vi "Test.vi"(0 "Call Context":T9, 5 "Test Controls":T3 {"Slider" scale=-1.0..1.0}) -> (1 "SubState 0":T2=enum."driver control", 2 "SubState 4":T2, 3 "Loop 0 Data":T7, 4 "SubState 1":T2, 6 "Loop 1 Data":T6, 10 "SubState 2":T2, 11 "SubState 5":T8, 12 "Loop 3 Data":T4, 13 "Loop 4 Data":T1, 14 "SubState 3":T2, 15 "Loop 2 Data":T5)   [LabVIEW 2013]
uses:
  typedefs/state machine/subStates.ctl
  <vilib>/Rock Robotics/WPI/DriverStation/WPI_DriverStationDerivedRobotMode.ctl
  typedefs/state machine/singleUseSubstate.ctl
  typedefs/loop datatypes/Loop 0 Datatype.ctl
  typedefs/loop datatypes/Loop 1 Datatype.ctl
  typedefs/loop datatypes/Loop 2 Datatype.ctl
  typedefs/loop datatypes/Loop 3 Datatype.ctl
  typedefs/test/test controls.ctl
  typedefs/loop datatypes/Loop 4 Datatype.ctl
  typedefs/fg_getset.ctl
  <vilib>/Rock Robotics/WPI/Joystick/WPI_JoystickGetSetRefNum.vi
panel:
  out "Compressor":bool
  out "JS Axis-Y 3":dbl
  out "JS Axis-X 3":dbl
  out "JS Axis-Y 2":dbl
  out "JS Axis-X 2":dbl
  out "UDB":bool
  out "JS Axis-X":dbl
  out "JS Axis-Y":dbl
  out "Exit Value":i32=-1
  # "Test Loop Data and Substates"
  # "Drive Loop"
  # "Loop 1"
  # "Loop 2"
  # "Loop 3"
  # "Loop 4"
  # "Pneumatics Loop"
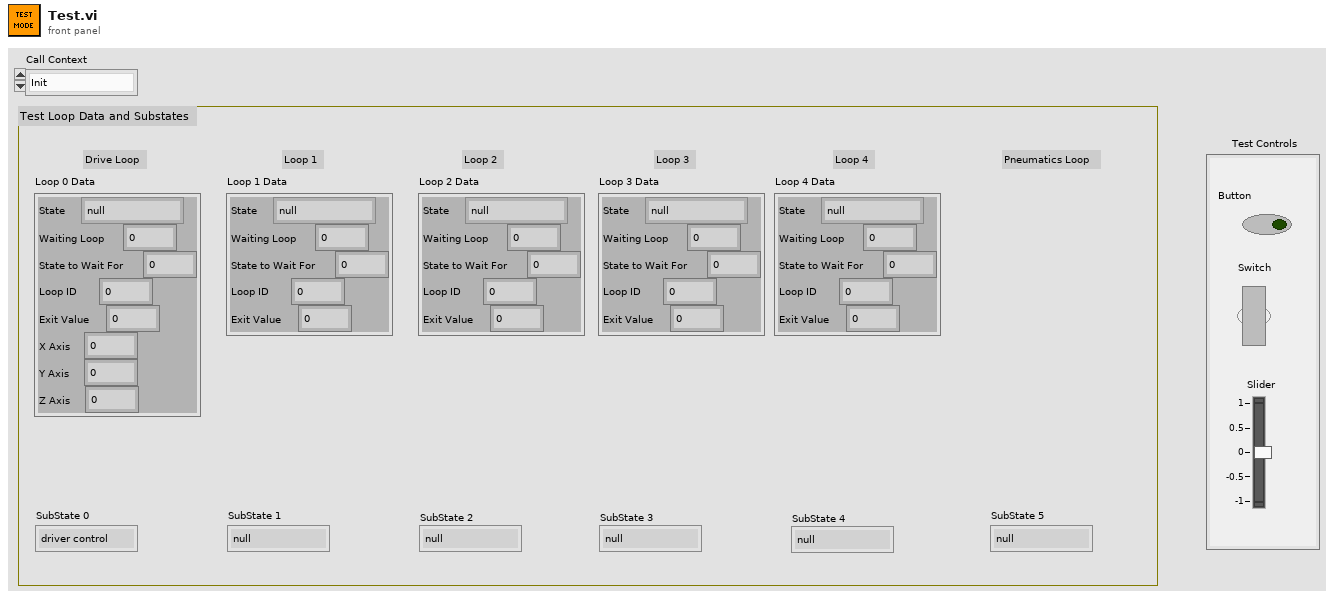
[diagram p1: front panel]
types:
  T1 = typedef "Loop 4 Datatype.ctl" = cluster{"State":T2, "Waiting Loop":i32, "State to Wait For":i32, "Loop ID":i32, "Exit Value":i32}
  T2 = typedef "subStates.ctl" = enum16{"null", "wait", "driver control", "auto", "manual override", "hold position", "rotate", "test", "end"}
  T3 = typedef "test controls.ctl" = cluster{"Button":bool, "Switch":bool, "Slider":dbl}
  T4 = typedef "Loop 3 Datatype.ctl" = cluster{"State":T2, "Waiting Loop":i32, "State to Wait For":i32, "Loop ID":i32, "Exit Value":i32}
  T5 = typedef "Loop 2 Datatype.ctl" = cluster{"State":T2, "Waiting Loop":i32, "State to Wait For":i32, "Loop ID":i32, "Exit Value":i32}
  T6 = typedef "Loop 1 Datatype.ctl" = cluster{"State":T2, "Waiting Loop":i32, "State to Wait For":i32, "Loop ID":i32, "Exit Value":i32}
  T7 = typedef "Loop 0 Datatype.ctl" = cluster{"State":T2, "Waiting Loop":i32, "State to Wait For":i32, "Loop ID":i32, "Exit Value":i32, "X Axis":dbl, "Y Axis":dbl, "Z Axis":dbl}
  T8 = typedef "singleUseSubstate.ctl" = enum16{"null", "wait", "shift high", "shift low", "end"}
  T9 = typedef "WPI_DriverStationDerivedRobotMode.ctl" = enum16{"Init", "Execute", "Stop"}
  T10 = typedef "fg_getset.ctl" = enum16{"Get", "Set"}
  T11 = typedef "WPI_JoystickDevRef.ctl" = cluster{"Device":T12}
  T12 = typedef "WPI_JoystickDeviceEnum.ctl" = enum16{"USB 1", "USB 2", "USB 3", "USB 4", "Kinect 1", "Kinect 2"}
  T13 = cluster{"axis 1 (x)":dbl, "axis 2 (y)":dbl, "axis 3 (throttle)":dbl, "axis 4":dbl, "axis 5":dbl, "axis 6":dbl}
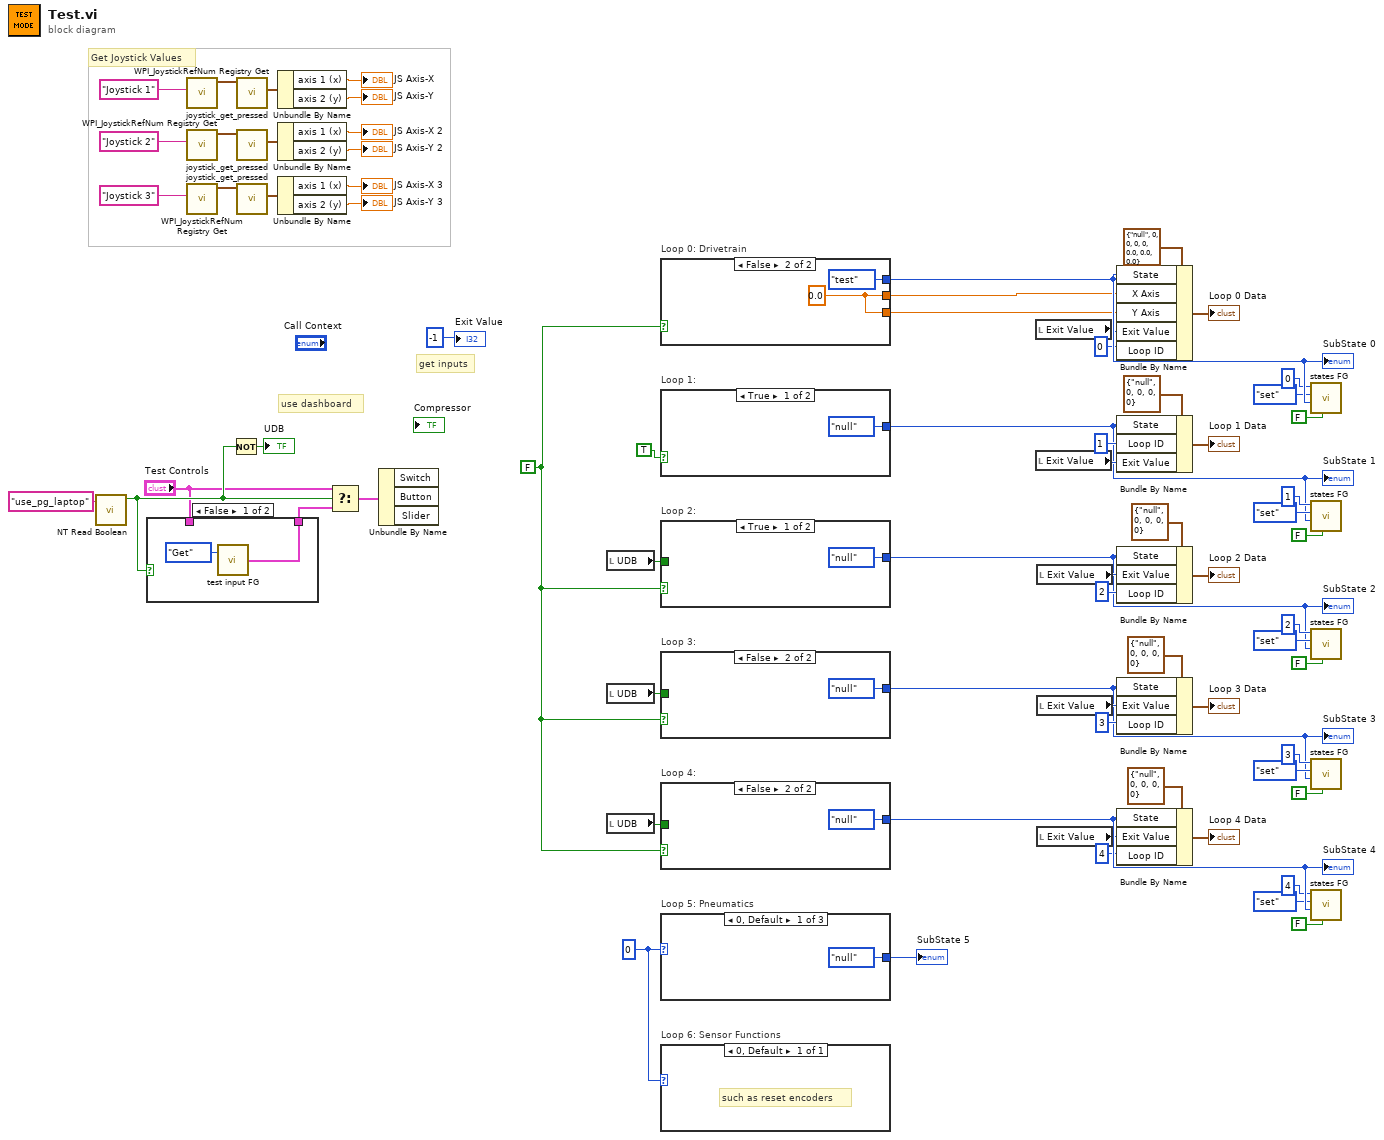
[diagram p0: block diagram]
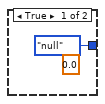
[diagram p2: hidden frame]
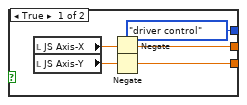
[diagram p4: hidden frame]
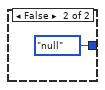
[diagram p5: hidden frame]
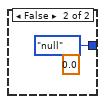
[diagram p6: hidden frame]
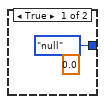
[diagram p7: hidden frame]
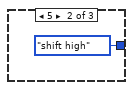
[diagram p8: hidden frame]
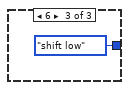
[diagram p9: hidden frame]
diagram:
  w1 = 0 ("Button Pressed")
  w6 = FALSE
  # "use dashboard"
  # "get inputs"
  # "Get Joystick Values"
  n1 = call <vilib>:"NT Read Boolean.vi"("Name"="use_pg_laptop") -> ("Boolean"=w31:bool)  [unwired: 9 in, 1 out]
  n2 = case shown="False" w31 {
    tunnel: [w73 w74] -> w29
    tunnel: "Test Controls" -> [_ w74]
    frame False {
      n3 = call "test input FG.vi"("Menu"=fg_getset."Get") -> ("Test Controls Out"=w73:T3)  [unwired: 1 in]
    }
    frame True {
    }
  }
  n4 = call <vilib>:"WPI_JoystickRefNum Registry Get.vi"("refnum name"="Joystick 1") -> ("JoystickDevRef"=w65:T11)  [unwired: 9 in, 1 out]
  n5 = call <vilib>:"WPI_JoystickRefNum Registry Get.vi"("refnum name"="Joystick 2") -> ("JoystickDevRef"=w25:T11)  [unwired: 9 in, 1 out]
  n6 = call <vilib>:"WPI_JoystickRefNum Registry Get.vi"("refnum name"="Joystick 3") -> ("JoystickDevRef"=w22:T11)  [unwired: 9 in, 1 out]
  n7 = Not(x=w31) -> (.not. x?=→"UDB":bool)
  n8 = call "joystick_get_pressed.vi"("JoystickDevRef"=w65) -> ("Axes"=w63:T13)  [unwired: 3 in, 3 out]
  n9 = call "joystick_get_pressed.vi"("JoystickDevRef"=w25) -> ("Axes"=w26:T13)  [unwired: 3 in, 3 out]
  n10 = call "joystick_get_pressed.vi"("JoystickDevRef"=w22) -> ("Axes"=w21:T13)  [unwired: 3 in, 3 out]
  n11 = Unbundle By Name(w63) -> ("axis 1 (x)"=→"JS Axis-X":dbl, "axis 2 (y)"=→"JS Axis-Y":dbl)
  n12 = Unbundle By Name(w26) -> ("axis 1 (x)"=→"JS Axis-X 2":dbl, "axis 2 (y)"=→"JS Axis-Y 2":dbl)
  n13 = Unbundle By Name(w21) -> ("axis 1 (x)"=→"JS Axis-X 3":dbl, "axis 2 (y)"=→"JS Axis-Y 3":dbl)
  n14 = Select(t="Test Controls", s=w31, f=w29) -> (s? t:f=w32:T3)
  n15 = Unbundle By Name(w32) -> ()  [unwired: 3 out]
  n16 = local read "UDB"() -> (w17:bool)
  n17 = local read "UDB"() -> (w16:bool)
  n18 = local read "UDB"() -> (w12:bool)
  n19 = case "Loop 0: Drivetrain" shown="False" w6 {
    tunnel: [w75 w80] -> w34
    tunnel: [subStates."driver control" ("State") subStates."test" ("State")] -> w71
    tunnel: [w76 w80] -> w35
    frame True {
      n20 = local read "JS Axis-X"() -> (w78:dbl)
      n21 = local read "JS Axis-Y"() -> (w77:dbl)
      n22 = Negate(x=w78) -> (-x=w76:dbl)
      n23 = Negate(x=w77) -> (-x=w75:dbl)
    }
    frame False {
      w80 = 0.0 ("JS Axis-X")
    }
  }
  "SubState 0" <- w71
  n24 = case "Loop 1:" shown="True" TRUE {
    tunnel: [subStates."null" ("State") subStates."null" ("State")] -> w42
    frame True {
    }
    frame False {
    }
  }
  "SubState 1" <- w42
  n25 = case "Loop 2:" shown="True" w6 {
    tunnel: [subStates."null" ("State") subStates."null" ("State")] -> w14
    tunnel: w17 -> [_ _]
    frame True {
    }
    frame False {
      (unwired) 0.0 ("Belts")
    }
  }
  "SubState 2" <- w14
  n26 = case "Loop 3:" shown="False" w6 {
    tunnel: [subStates."null" ("State") subStates."null" ("State")] -> w15
    tunnel: w16 -> [_ _]
    frame True {
      (unwired) 0.0 ("Arm")
    }
    frame False {
    }
  }
  "SubState 3" <- w15
  n27 = case "Loop 4:" shown="False" w6 {
    tunnel: [subStates."null" ("State") subStates."null" ("State")] -> w13
    tunnel: w12 -> [_ _]
    frame True {
      (unwired) 0.0 ("Arm")
    }
    frame False {
    }
  }
  "SubState 4" <- w13
  n28 = case "Loop 5: Pneumatics" shown="0, Default" w1 {
    tunnel: [singleUseSubstate."null" ("SubState 4") singleUseSubstate."shift high" ("SubState 4") singleUseSubstate."shift low" ("SubState 4")] -> w70
    frame 0, Default {
    }
    frame 5 {
    }
    frame 6 {
    }
  }
  "SubState 5" <- w70
  n29 = case "Loop 6: Sensor Functions" shown="0, Default" w1 {
    frame 0, Default {
      # "such as reset encoders"
    }
  }
  n30 = local read "Exit Value"() -> (w39:i32)
  n31 = local read "Exit Value"() -> (w50:i32)
  n32 = local read "Exit Value"() -> (w54:i32)
  n33 = local read "Exit Value"() -> (w64:i32)
  n34 = local read "Exit Value"() -> (w7:i32)
  n35 = Bundle By Name(cluster=T7 {"State"=enum."null", "Waiting Loop"=0, "State to Wait For"=0, "Loop ID"=0, "Exit Value"=0, "X Axis"=0.0, "Y Axis"=0.0, "Z Axis"=0.0} ("Loop 0 Data"), "State"=w71, "X Axis"=w35, "Y Axis"=w34, "Exit Value"=w39, "Loop ID"=0) -> (→"Loop 0 Data":T7)
  n36 = Bundle By Name(cluster=T6 {"State"=enum."null", "Waiting Loop"=0, "State to Wait For"=0, "Loop ID"=0, "Exit Value"=0} ("Loop 1 Data"), "State"=w42, "Loop ID"=1, "Exit Value"=w50) -> (→"Loop 1 Data":T6)
  n37 = Bundle By Name(cluster=T5 {"State"=enum."null", "Waiting Loop"=0, "State to Wait For"=0, "Loop ID"=0, "Exit Value"=0} ("Loop 2 Data"), "State"=w14, "Exit Value"=w54, "Loop ID"=2) -> (→"Loop 2 Data":T5)
  n38 = Bundle By Name(cluster=T4 {"State"=enum."null", "Waiting Loop"=0, "State to Wait For"=0, "Loop ID"=0, "Exit Value"=0} ("Loop 3 Data"), "State"=w15, "Exit Value"=w64, "Loop ID"=3) -> (→"Loop 3 Data":T4)
  n39 = Bundle By Name(cluster=T1 {"State"=enum."null", "Waiting Loop"=0, "State to Wait For"=0, "Loop ID"=0, "Exit Value"=0} ("Loop 4 Data"), "State"=w13, "Exit Value"=w7, "Loop ID"=4) -> (→"Loop 4 Data":T1)
  n40 = call "states FG.vi"("exit in"=FALSE, "subState in"=w71, "menu (get)"=enum16{"set", "get"}."set", "Loop ID"=0) -> ()  [unwired: 4 in, 4 out]
  n41 = call "states FG.vi"("exit in"=FALSE, "subState in"=w42, "menu (get)"=enum16{"set", "get"}."set", "Loop ID"=1) -> ()  [unwired: 4 in, 4 out]
  n42 = call "states FG.vi"("exit in"=FALSE, "subState in"=w14, "menu (get)"=enum16{"set", "get"}."set", "Loop ID"=2) -> ()  [unwired: 4 in, 4 out]
  n43 = call "states FG.vi"("exit in"=FALSE, "subState in"=w15, "menu (get)"=enum16{"set", "get"}."set", "Loop ID"=3) -> ()  [unwired: 4 in, 4 out]
  n44 = call "states FG.vi"("exit in"=FALSE, "subState in"=w13, "menu (get)"=enum16{"set", "get"}."set", "Loop ID"=4) -> ()  [unwired: 4 in, 4 out]
  "Exit Value" <- -1 ("Exit Value")
